vi "ShowClassPanMessage.vi"(8 "ErrorIn(NoErr)":errorcluster caption="entrée d'erreur (pas d'erreur)", 10 "Tableau":string[](array[string]), 11 "Show All":bool) -> (0 "ErrorOut(NoErr)":errorcluster caption="entrée d'erreur (pas d'erreur)", 3 "Show":bool[](array[boolean]))   [LabVIEW 2019]
panel:
  in  "Quit":bool
  in  "ShowPanels":cluster{"Name":string, "Show":bool}[](array[cluster])
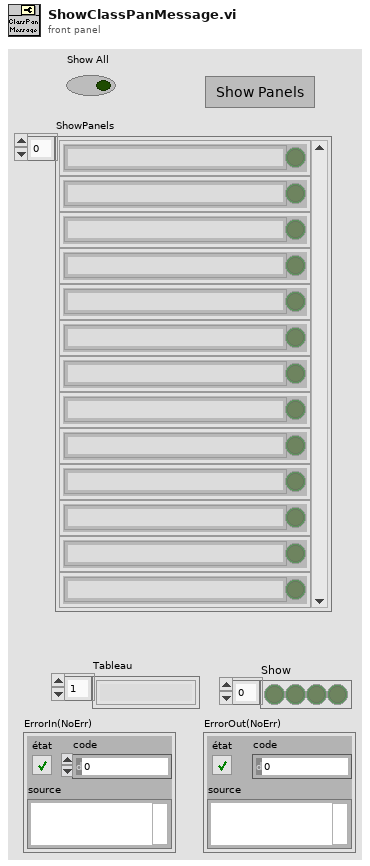
[diagram p1: front panel]
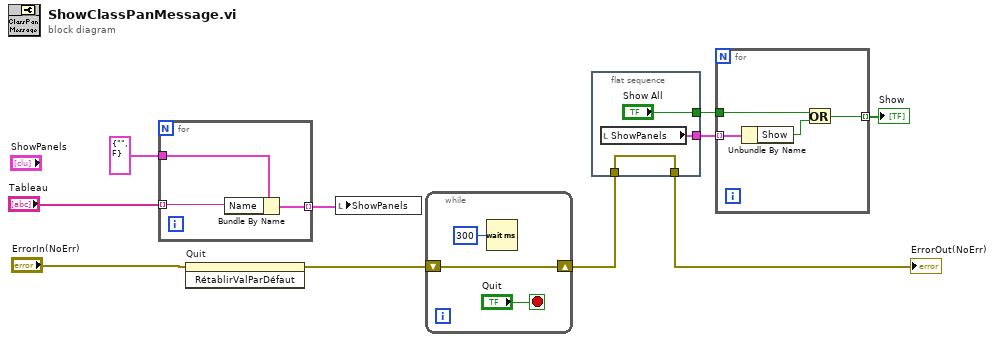
[diagram p0: block diagram]
diagram:
  n1 = for {
    tunnel: "Tableau" -> [w12] mode=indexing
    tunnel: cluster{"Name":string, "Show":bool} {"Name"="", "Show"=FALSE} ("ShowPanel") -> [w13]
    tunnel: [w11] -> w6 mode=indexing
    n2 = Bundle By Name(cluster=w13, "Name"=w12) -> (w11:cluster{"Name":string, "Show":bool})
  }
  n3 = invoke on="Quit" class="Bool" method="RétablirValParDéfaut"(error in="ErrorIn(NoErr)") -> (error out=w7:errorcluster)  [unwired: 2 in, 2 out]
  n4 = local write "ShowPanels"(w6) -> ()
  n5 = while {
    shift-right: [w14] -> w4
    shift-left: w7 -> [w14]
    stop <- "Quit" stop-if-true
    n6 = Wait (ms)(milliseconds to wait=u32 300 ("attente (ms)")) -> ()  [unwired: 1 out]
  }
  n7 = flat-sequence {
    tunnel: [w19] -> w5
    tunnel: [w18] -> w3
    tunnel: w4 -> [w18]
    tunnel: ["Show All"] -> w2
    frame #0 {
      n8 = local read "ShowPanels"() -> (w19:cluster{"Name":string, "Show":bool}[])
    }
  }
  n9 = for {
    tunnel: w2 -> [w23]
    tunnel: w5 -> [w22] mode=indexing
    tunnel: [w20] -> w1 mode=indexing
    n10 = Unbundle By Name(w22) -> ("Show"=w21:bool)
    n11 = Or(x=w23, y=w21) -> (x .or. y?=w20:bool)
  }
  "Show" <- w1
  "ErrorOut(NoErr)" <- w3
